vi "Configure Number of Averages [AA] Core.vi"(8 "error in (no error)":errorcluster, 10 "number of averages (8)":i32=8, 11 "CS++Scope":refnum<class "CS++Scope.lvclass">) -> (0 "error out":errorcluster, 3 "CS++Scope out":refnum<class "CS++Scope.lvclass">)   [LabVIEW 2013, in "CS++Scope.lvlib" / "CS++Scope.lvclass"]
doc: "When you set the acquisition type to IVISCOPE_VAL_AVERAGE, the oscilloscope acquires multiple waveforms. After each waveform acquisition, the oscilloscope keeps the average value of all acquisitions for each element in the waveform record. This VI configures the number of waveforms that the oscilloscope acquires and averages. After the oscilloscope acquires as many waveforms as you specify, it returns to the idle state."
uses:
  CS++Scope.lvclass
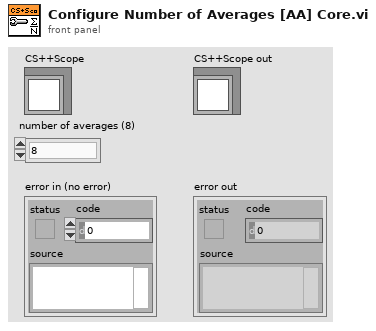
[diagram p1: front panel]
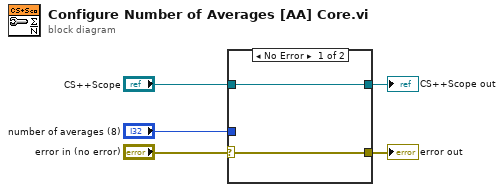
[diagram p0: block diagram]
diagram:
  n1 = case shown="No Error" "error in (no error)" {
    selector: "error in (no error)" -> [w6 w9]
    tunnel: [w6 w9] -> w4
    tunnel: [w7 w8] -> w2
    tunnel: "CS++Scope" -> [w7 w8]
    tunnel: "number of averages (8)" -> [_ _]
    frame No Error {
    }
    frame Error {
    }
  }
  "error out" <- w4
  "CS++Scope out" <- w2
